vi "Caculate.vi"(6 "Enum":T1, 8 "error in (no error)":errorcluster, 9 "b":dbl, 10 "a":dbl, 11 "Cacluator in":refnum<class "Cacluator.lvclass">) -> (0 "error out":errorcluster, 2 "Result":dbl, 3 "Cacluator out":refnum<class "Cacluator.lvclass">)   [LabVIEW 2014, in "Caculator.lvlib" / "Cacluator.lvclass"]
uses:
  Cacluator.lvclass
  Enum.ctl
  Strategy_class/Strategy.lvclass
  Caculator.lvlib
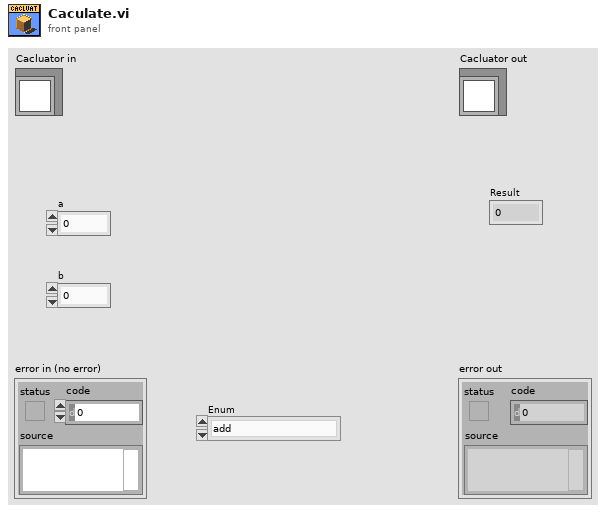
[diagram p1: front panel]
types:
  T1 = typedef "Caculator.lvlib/Enum.ctl" = enum16{"add", "subtract"}
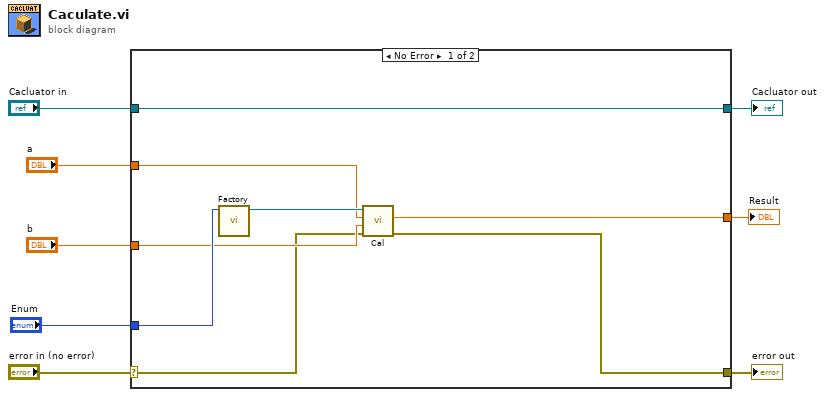
[diagram p0: block diagram]
diagram:
  n1 = case shown="No Error" "error in (no error)" {
    selector: "error in (no error)" -> [w11 w18]
    tunnel: [w10 w18] -> w7
    tunnel: [w16 w17] -> w5
    tunnel: "Cacluator in" -> [w16 w17]
    tunnel: "Enum" -> [w15 _]
    tunnel: "a" -> [w13 _]
    tunnel: "b" -> [w12 _]
    tunnel: [w9 _] -> w1
    frame No Error {
      n2 = call "Factory.vi"("Enum"=w15) -> ("Caculator.lvlib:Strategy"=w14:refnum<class "Strategy.lvclass">)  [unwired: 10 in]
      n3 = call-dynamic "Cal.vi"("error in (no error)"=w11, "b"=w12, "a"=w13, "Strategy in"=w14) -> ("error out"=w10:errorcluster, "Result"=w9:dbl)  [unwired: 5 in, 1 out]
    }
    frame Error {
    }
  }
  "error out" <- w7
  "Cacluator out" <- w5
  "Result" <- w1
